vi "SWITCH_MOVE.vi"(8 "RESET":bool, 11 "ARM 1 & 2 INPUTS":T1) -> (0 "ARM 2 SETPOINT OUT":dbl, 2 "RUNNING?":bool, 3 "ARM 1 SETPOINT OUT":dbl)   [LabVIEW 2017]
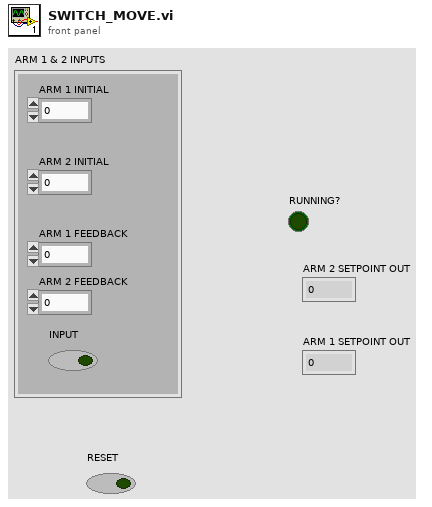
[diagram p1: front panel]
types:
  T1 = cluster{"ARM 1 INITIAL":dbl, "ARM 2 INITIAL":dbl, "ARM 1 FEEDBACK":dbl, "ARM 2 FEEDBACK":dbl, "INPUT":bool}
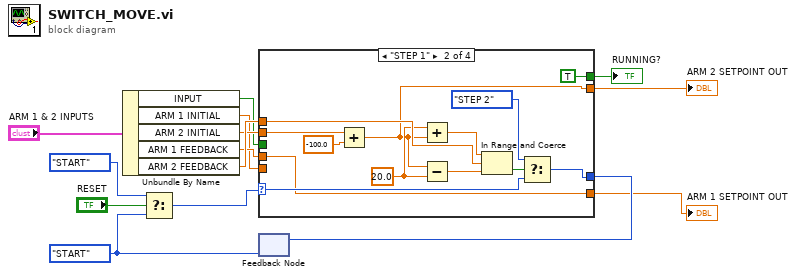
[diagram p0: block diagram]
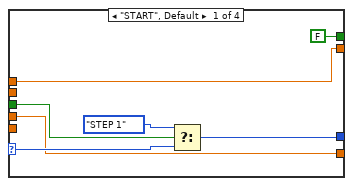
[diagram p2: hidden frame]
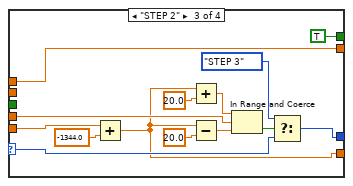
[diagram p3: hidden frame]
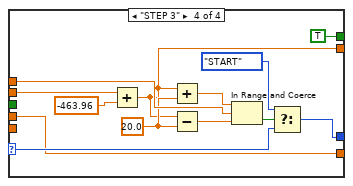
[diagram p4: hidden frame]
diagram:
  w2 = enum16{"START", "STEP 1", "STEP 2", "STEP 3"}."START"
  n1 = Unbundle By Name("ARM 1 & 2 INPUTS") -> ("INPUT"=w5:bool, "ARM 1 INITIAL"=w6:dbl, "ARM 2 INITIAL"=w7:dbl, "ARM 1 FEEDBACK"=w8:dbl, "ARM 2 FEEDBACK"=w9:dbl)
  n2 = Select(t=enum16{"START", "STEP 1", "STEP 2", "STEP 3"}."START", s="RESET", f=w2) -> (s? t:f=w3:enum16{"START", "STEP 1", "STEP 2", "STEP 3"})
  n3 = case shown="\"STEP 1\"" w3 {
    selector: w3 -> [w20 w34 w48 w61]
    tunnel: [w21 w33 w47 w60] -> w14
    tunnel: w5 -> [w19 _ _ _]
    tunnel: w6 -> [_ _ w37 _]
    tunnel: w7 -> [_ w26 _ w50]
    tunnel: w9 -> [w16 w27 w35 w55]
    tunnel: [w16 w22 w35 w49] -> w13
    tunnel: w8 -> [w17 w30 w39 w58]
    tunnel: [w17 w30 w36 w58] -> w12
    tunnel: [FALSE TRUE TRUE TRUE] -> w11
    frame "START", Default {
      n4 = Select(t=enum16{"START", "STEP 1", "STEP 2", "STEP 3"}."STEP 1", s=w19, f=w20) -> (s? t:f=w21:enum16{"START", "STEP 1", "STEP 2", "STEP 3"})
    }
    frame "STEP 1" {
      w23 = 20.0 ("x")
      n5 = Add(x=w26, y=-100.0) -> (x+y=w22:dbl)
      n6 = Add(x=w23, y=w22) -> (x+y=w24:dbl)
      n7 = Subtract(x=w22, y=w23) -> (x-y=w25:dbl)
      n8 = In Range and Coerce(upper limit=w24, x=w27, lower limit=w25) -> (In Range?=w28:bool)  [unwired: 1 out]
      n9 = Select(t=enum16{"START", "STEP 1", "STEP 2", "STEP 3"}."STEP 2", s=w28, f=w34) -> (s? t:f=w33:enum16{"START", "STEP 1", "STEP 2", "STEP 3"})
    }
    frame "STEP 2" {
      n10 = Add(x=w37, y=-1344.0) -> (x+y=w36:dbl)
      n11 = Add(x=w36, y=20.0) -> (x+y=w43:dbl)
      n12 = Subtract(x=w36, y=20.0) -> (x-y=w42:dbl)
      n13 = In Range and Coerce(upper limit=w43, x=w39, lower limit=w42) -> (In Range?=w44:bool)  [unwired: 1 out]
      n14 = Select(t=enum16{"START", "STEP 1", "STEP 2", "STEP 3"}."STEP 3", s=w44, f=w48) -> (s? t:f=w47:enum16{"START", "STEP 1", "STEP 2", "STEP 3"})
    }
    frame "STEP 3" {
      w52 = 20.0 ("y")
      n15 = Add(x=w50, y=-463.96) -> (x+y=w49:dbl)
      n16 = Add(x=w49, y=w52) -> (x+y=w53:dbl)
      n17 = Subtract(x=w49, y=w52) -> (x-y=w54:dbl)
      n18 = In Range and Coerce(upper limit=w53, x=w55, lower limit=w54) -> (In Range?=w56:bool)  [unwired: 1 out]
      n19 = Select(t=enum16{"START", "STEP 1", "STEP 2", "STEP 3"}."START", s=w56, f=w61) -> (s? t:f=w60:enum16{"START", "STEP 1", "STEP 2", "STEP 3"})
    }
  }
  "ARM 2 SETPOINT OUT" <- w13
  "ARM 1 SETPOINT OUT" <- w12
  "RUNNING?" <- w11
  n20 = feedback-in #1(w14) -> ()
  n21 = feedback #1(w2) -> ()  [unwired: 1 in]
